vi "_Insert SubPanel.vi"(8 "error in (no error)":errorcluster, 9 "VI Refnum":refnum<vi>, 10 "Index":i32, 11 "Item_Refnums_Array":T1[](array[typedef])) -> (0 "error out":errorcluster, 3 "Item_Refnums_Array Out":T1[](array[typedef]))   [LabVIEW 2013, in "UI Panels.lvlib" / "Panels_XControl.xctl"]
uses:
  Panels_XControl.xctl
  Controls/References/Panel_Refnums.ctl
  Controls/Panel_Command_Enum.ctl
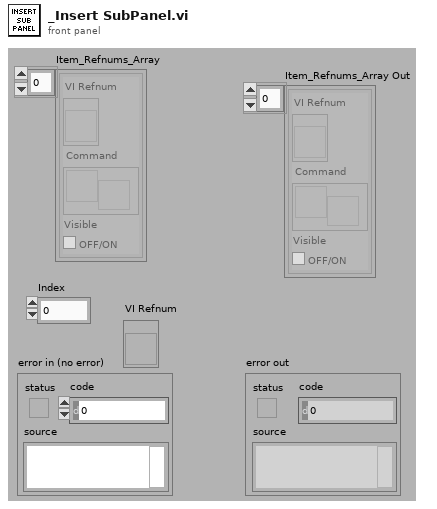
[diagram p1: front panel]
types:
  T1 = typedef "UI Panels.lvlib/Panels_XControl.xctl/Panel_Refnums.ctl" = cluster{"VI Refnum":refnum<vi>, "Command":refnum<user-event>, "Visible":bool}
  T2 = typedef "UI Panels.lvlib/Panels_XControl.xctl/Panel_Command_Enum.ctl" = enum16{"Idle", "Remove & Stop", "Add Item", "Delete Item", "Delete All", "Insert into Subpanel", "Register Menu Events", "Update Value", "Remove from Subpanel", "Set Title", "Set Menu Items", "Insert SubPanel", "Set Splitter Position", "Set Splitter Properties", "Add Menu Items"}
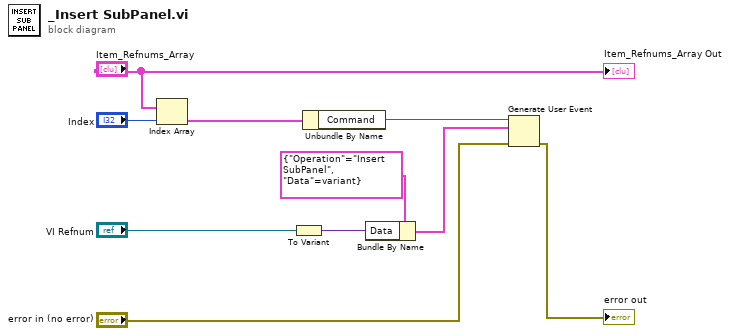
[diagram p0: block diagram]
diagram:
  n1 = Index Array(array="Item_Refnums_Array", index="Index") -> (element=w7:T1)
  n2 = To Variant(anything="VI Refnum") -> (Variant=w5:variant)
  n3 = Unbundle By Name(w7) -> ("Command"=w4:refnum<user-event>)
  n4 = Bundle By Name(cluster=cluster{"Operation":T2, "Data":variant} {"Operation"=enum."Insert SubPanel", "Data"=variant} ("Item_Command"), "Data"=w5) -> (w3:cluster{"Operation":T2, "Data":variant})
  n5 = Generate User Event(user event=w4, event data cluster=w3, error in="error in (no error)") -> (error out=→"error out":errorcluster)  [unwired: 1 in, 1 out]
  "Item_Refnums_Array Out" <- "Item_Refnums_Array"
